vi "MSScript_Exe_Cmd_IfFalse.vi"(5 "Index":i32, 6 "error in (no error)":errorcluster, 7 "End":string, 8 "Start":string, 9 "MSScript in":refnum<class "MSScript.lvclass">) -> (0 "Error out":errorcluster, 3 "Index of the next sentence":i32)   [LabVIEW 2018, in "MSScript.lvclass"]
uses:
  MSScript.lvclass
  MSScript.lvclass/MSScript.ctl
  MSScript_Error_(6010)CommentLost.vi
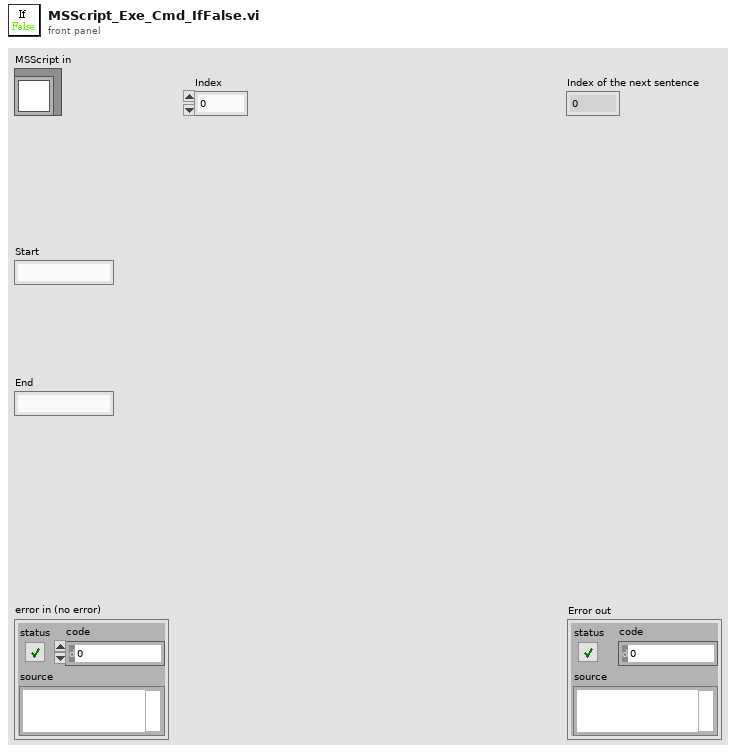
[diagram p1: front panel]
types:
  T1 = cluster{"Type":string, "NAME":cluster{"STR":string, "Start":i32}, "PARAMs":cluster{"STR":string, "Start":i32}[]}[]
  T2 = cluster{"Type":string, "NAME":cluster{"STR":string, "Start":i32}, "PARAMs":cluster{"STR":string, "Start":i32}[]}
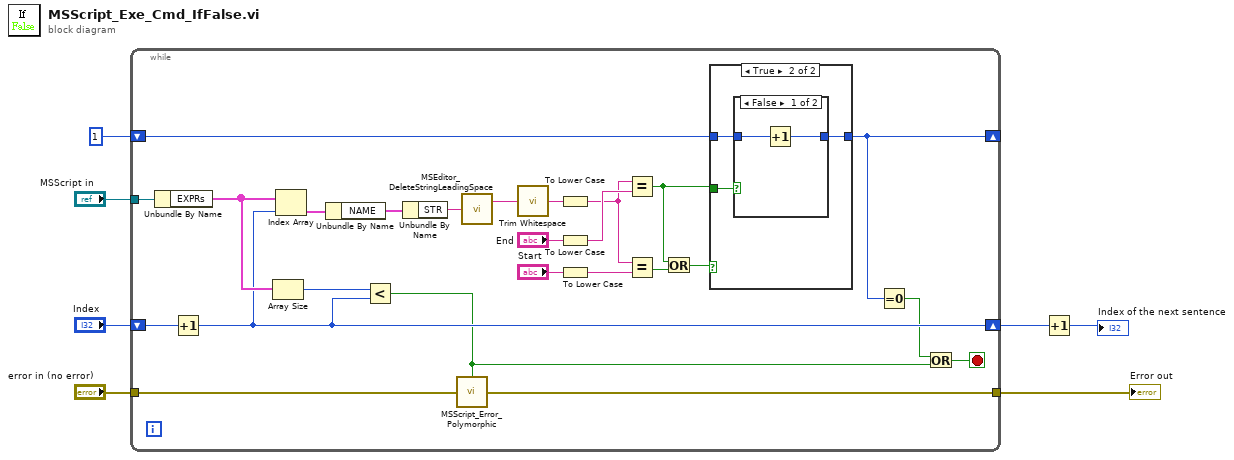
[diagram p0: block diagram]
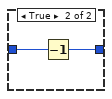
[diagram p3: hidden frame]
diagram:
  n1 = while {
    tunnel: "MSScript in" -> [w32]
    shift-right: [w24] -> w2
    shift-left: "Index" -> [w29]
    shift-right: [w15] -> _
    shift-left: 1 -> [w16]
    tunnel: "error in (no error)" -> [w13]
    tunnel: [w12] -> w3
    stop <- w23 stop-if-true
    n2 = Unbundle By Name(w32) -> ("EXPRs"=w26:T1)
    n3 = Increment(x=w29) -> (x+1=w24:i32)
    n4 = Array Size(array=w26) -> (size(s)=w25:i32)
    n5 = Index Array(array=w26, index=w24) -> (element=w31:T2)
    n6 = Unbundle By Name(w31) -> ("NAME"=w30:cluster{"STR":string, "Start":i32})
    n7 = Less?(x=w25, y=w24) -> (x < y?=w22:bool)
    n8 = Unbundle By Name(w30) -> ("STR"=w27:string)
    n9 = call-poly "MSScript_Error_Polymorphic.vi"("error in (no error)"=w13, "ErrBoolean"=w22) -> ("error out"=w12:errorcluster)
    n10 = call "MSEditor_DeleteStringLeadingSpace.vi"("string in"=w27) -> ("string after leading space"=w28:string)  [unwired: 1 out]
    n11 = call <vilib>:"Trim Whitespace.vi"("string"=w28) -> ("trimmed string"=w20:string)  [unwired: 1 in]
    n12 = To Lower Case(string=w20) -> (all lower case string=w8:string)
    n13 = To Lower Case(string="End") -> (all lower case string=w9:string)
    n14 = To Lower Case(string="Start") -> (all lower case string=w10:string)
    n15 = Equal?(x=w8, y=w9) -> (x = y?=w17:bool)
    n16 = Equal?(x=w8, y=w10) -> (x = y?=w19:bool)
    n17 = Or(x=w17, y=w19) -> (x .or. y?=w18:bool)
    n18 = case shown="True" w18 {
      tunnel: w17 -> [_ w34]
      tunnel: w16 -> [w33 w36]
      tunnel: [w33 w35] -> w15
      frame False {
      }
      frame True {
        n19 = case shown="False" w34 {
          tunnel: w36 -> [w38 w40]
          tunnel: [w37 w39] -> w35
          frame False {
            n20 = Increment(x=w38) -> (x+1=w37:i32)
          }
          frame True {
            n21 = Decrement(x=w40) -> (x-1=w39:i32)
          }
        }
      }
    }
    n22 = Equal To 0?(x=w15) -> (x = 0?=w14:bool)
    n23 = Or(x=w14, y=w22) -> (x .or. y?=w23:bool)
  }
  "Error out" <- w3
  n24 = Increment(x=w2) -> (x+1=→"Index of the next sentence":i32)
